vi "SetGUILanguage.vi"(0 "Lang file path":path, 2 "viPath":path) -> ()   [LabVIEW 2020]
doc: "Set vi language with the localized ini language file."
uses:
  <vilib>/Utility/config.llb/Read Key (String).vi
  <vilib>/Utility/config.llb/NI_LVConfig.lvlib
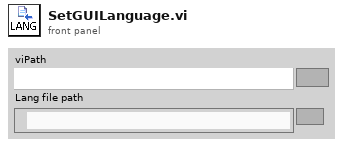
[diagram p1: front panel]
types:
  T1 = typedef "NI_LVConfig.lvlib/Config Data RefNum.ctl" = refnum<k1>
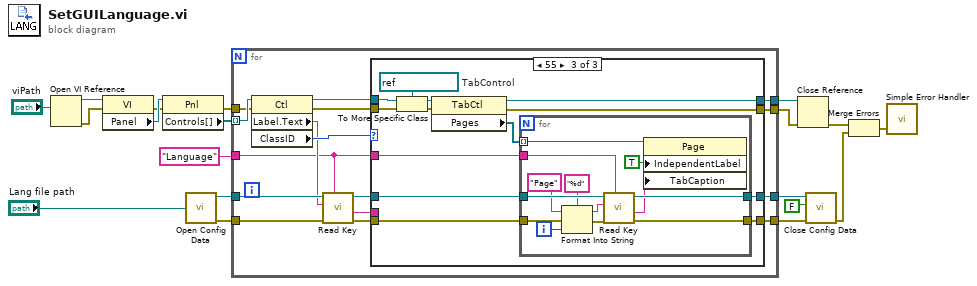
[diagram p0: block diagram]
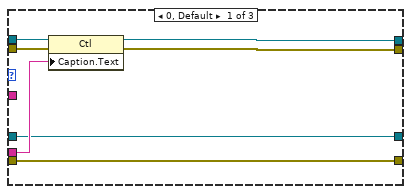
[diagram p2: hidden frame]
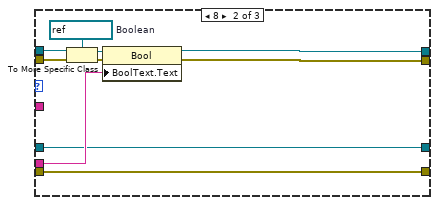
[diagram p3: hidden frame]
diagram:
  n1 = Open VI Reference(vi path="viPath") -> (vi reference=w13:refnum<vi>, error out=w12:errorcluster)  [unwired: 2 in, 3 out]
  n2 = property class="VI"(reference=w13, error in=w12) -> (error out=w18:errorcluster, "Panel"=w19:refnum<vi>)  [unwired: 1 out]
  n3 = property class="Pnl"(reference=w19, error in=w18) -> (error out=w16:errorcluster, "Controls[]"=w17:refnum<vi>[])  [unwired: 1 out]
  n4 = call <vilib>:"Open Config Data.vi"("configuration file path"="Lang file path") -> ("error out"=w8:errorcluster, "refnum"=w9:T1)  [unwired: 8 in, 1 out]
  n5 = for {
    tunnel: w17 -> [w35] mode=indexing
    tunnel: w9 -> [w28]
    tunnel: w8 -> [w27]
    tunnel: w16 -> [w34]
    tunnel: [w31] -> w15
    tunnel: [w30] -> w14
    tunnel: "Language" ("name") -> [w21]
    tunnel: [w23] -> w6
    tunnel: [w20] -> w5
    n6 = property class="Ctl"(reference=w35, error in=w34) -> (reference out=w33:refnum<vi>, error out=w32:errorcluster, "Label.Text"=w25:string, "ClassID"=w29:u32)
    n7 = call-poly <vilib>:"Read Key.vi"("section"=w21, "error in (no error)"=w27, "key"=w25, "refnum"=w28) -> ("error out"=w22:errorcluster, "value"=w26:string, "refnum out"=w24:T1)  [unwired: 2 in, 3 out]
    n8 = case shown="55" w29 {
      tunnel: w33 -> [w41 w48 w63]
      tunnel: w32 -> [w42 w51 w64]
      tunnel: [w38 w46 w65] -> w31
      tunnel: [w39 w47 w59] -> w30
      tunnel: w26 -> [w40 w45 _]
      tunnel: w24 -> [w36 w44 w57]
      tunnel: [w36 w44 w56] -> w23
      tunnel: w22 -> [w37 w43 w54]
      tunnel: w21 -> [_ _ w55]
      tunnel: [w37 w43 w53] -> w20
      frame 0, Default {
        n9 = property class="Ctl"(reference=w41, error in=w42, "Caption.Text"=w40) -> (reference out=w39:refnum<vi>, error out=w38:errorcluster)
      }
      frame 8 {
        w52 = refnum<vi> refnum  # Boolean
        n10 = To More Specific Class(target class=w52, reference=w48, error in=w51) -> (specific class reference=w49:refnum<vi>, error out=w50:errorcluster)
        n11 = property class="Bool"(reference=w49, error in=w50, "BoolText.Text"=w45) -> (reference out=w47:refnum<vi>, error out=w46:errorcluster)
      }
      frame 55 {
        w60 = refnum<vi> refnum  # TabControl
        n12 = To More Specific Class(target class=w60, reference=w63, error in=w64) -> (specific class reference=w62:refnum<vi>, error out=w61:errorcluster)
        n13 = property class="TabCtl"(reference=w62, error in=w61) -> (reference out=w59:refnum<vi>, error out=w65:errorcluster, "Pages"=w58:refnum<vi>[])
        n14 = for {
          tunnel: w58 -> [w78] mode=indexing
          tunnel: w57 -> [w76]
          tunnel: [w75] -> w56
          tunnel: w55 -> [w69]
          tunnel: w54 -> [w68]
          tunnel: [w66] -> w53
          i -> [w73]
          n15 = Format Into String(format string="%d", initial string="Page", error in=w68, w73) -> (resulting string=w70:string, error out=w67:errorcluster)
          n16 = call-poly <vilib>:"Read Key.vi"("section"=w69, "error in (no error)"=w67, "key"=w70, "refnum"=w76) -> ("error out"=w66:errorcluster, "value"=w74:string, "refnum out"=w75:T1)  [unwired: 2 in, 3 out]
          n17 = property class="Page"(reference=w78, "IndependentLabel"=TRUE ("Independent Label"), "TabCaption"=w74) -> ()  [unwired: 1 in, 2 out]
        }
      }
    }
  }
  n18 = Close Reference(reference=w14, error in (no error)=w15) -> (error out=w3:errorcluster)
  n19 = call <vilib>:"Close Config Data.vi"("error in (no error)"=w5, "write file if changed (T)"=FALSE ("write configuration file? (T)"), "refnum"=w6) -> ("error out"=w2:errorcluster)  [unwired: 8 out]
  n20 = Merge Errors(w3, w2) -> (w1:errorcluster)
  n21 = call <vilib>:"Simple Error Handler.vi"("error in (no error)"=w1) -> ()  [unwired: 1 in, 8 out]
